vi "WPI_I2CReadOnly.vi"(8 "error in (no error)":errorcluster, 9 "I2CBytesToRead":u8, 11 "I2CDevRef":T1={"DevStatus"={"status"=FALSE, "code"=0, "source"=""}, "Device Address"=0, "Handle"=0, "I2C Bus"=enum."Invalid"} {"Device Address" format="%.0x"}) -> (0 "error out":errorcluster, 2 "Data Out":u8[](array[numeric]), 3 "I2CDevRef":T1={"DevStatus"={"status"=FALSE, "code"=0, "source"=""}, "Device Address"=0, "Handle"=0, "I2C Bus"=enum."Invalid"} {"Device Address" format="%.0x"})   [LabVIEW 2015]
doc: "Reads between one and four bytes in a single transaction from the I2C sensor you specify.\n\nThis software is licensed. Open the labview\\readme\\WPI Robotics Library Open Source License.txt file for more information."
uses:
  <vilib>/Rock Robotics/WPI/I2C/WPI_I2CDevRef.ctl
  <vilib>/Rock Robotics/SystemInterfaces/i2clib/i2c_bus.ctl
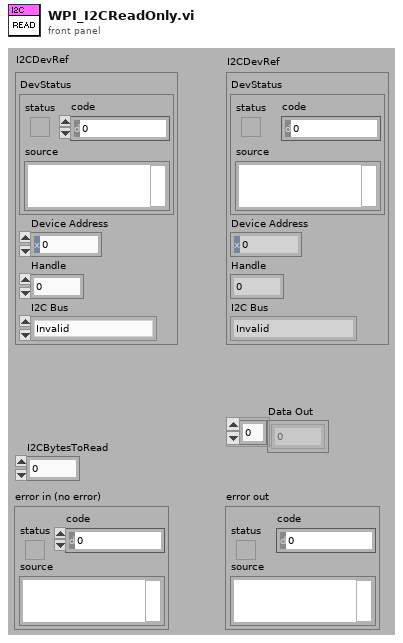
[diagram p1: front panel]
types:
  T1 = typedef "WPI_I2CDevRef.ctl" = cluster{"DevStatus":errorcluster, "Device Address":u8, "Handle":i32, "I2C Bus":T2}
  T2 = typedef "i2c_bus.ctl" = enum16{"I2C On-Board", "I2C MXP", "Invalid"}
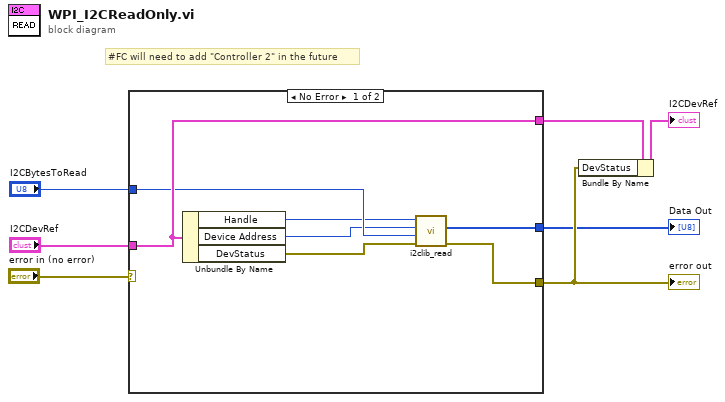
[diagram p0: block diagram]
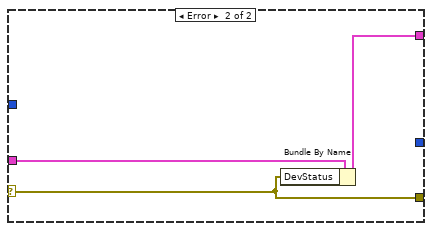
[diagram p2: hidden frame]
diagram:
  # "#FC will need to add \"Controller 2\" in the future"
  n1 = case shown="No Error" "error in (no error)" {
    selector: "error in (no error)" -> [_ w15]
    tunnel: [w9 w15] -> w2
    tunnel: "I2CDevRef" -> [w14 w17]
    tunnel: [w14 w16] -> w4
    tunnel: "I2CBytesToRead" -> [w13 _]
    tunnel: [w8 _] -> w1
    frame No Error {
      n2 = Unbundle By Name(w14) -> ("Handle"=w11:i32, "Device Address"=w10:u8, "DevStatus"=w12:errorcluster)
      n3 = call <vilib>:"i2clib_read.vi"("error in (no error)"=w12, "recv_size"=w13, "dev_addr"=w10, "I2C Reference"=w11) -> ("error out"=w9:errorcluster, "recv_data"=w8:u8[])  [unwired: 5 in, 1 out]
    }
    frame Error {
      n4 = Bundle By Name(cluster=w17, "DevStatus"=w15) -> (w16:T1)
    }
  }
  "error out" <- w2
  "Data Out" <- w1
  n5 = Bundle By Name(cluster=w4, "DevStatus"=w2) -> (→"I2CDevRef":T1)
